vi "Engine-DI-Run.vi"(8 "Error In":errorcluster, 11 "DSI Reference":refnum<class "DCM-DSI.lvclass">) -> (0 "Error Out":errorcluster, 3 "DSI Reference":refnum<class "DCM-DSI.lvclass">)   [LabVIEW 2016, in "DSI-RT.lvlib"]
uses:
  DSI-RT.lvlib
  Classes/DCM-DSI/DCM-DSI.lvclass
  Classes/DCM-DSI/Read DI-A Command.vi
  Classes/DCM-DSI/Read DI-B Command.vi
  Classes/DCM-DSI/Read Channels.vi
  Classes/DCM-DSI/Write DI-A Command.vi
  Classes/DCM-DSI/Write DI-B Command.vi
  Classes/DCM-DSI/Write Channels.vi
  <vilib>/addons/Software Calibration Management/xSCM/CalPoint.xnode
  <vilib>/addons/Software Calibration Management/xSCM/FaultPoint.xnode
  <vilib>/addons/Software Calibration Management/xSCM/ni_scm.dll
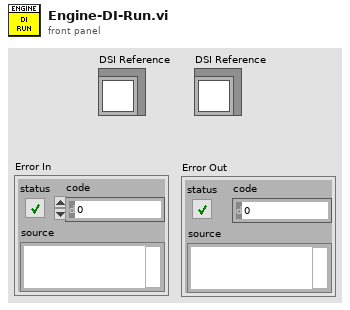
[diagram p1: front panel]
types:
  T1 = typedef "DCM - RT - DI.lvlib/Command.ctl" = cluster{"Mode":T2, "Digital Input":T3, "Default Profile Index":u8, "Cal Freq [Hz]":sgl, "Cal Duration [s]":sgl, "Cal Increment [s]":sgl, "Cal Pulses":u16, "TMP Command Sequence":T4[], "EPT TDC Offset [CAD]":sgl, "EPT Window Start [DBTDC]":sgl, "EPT Window End [DBTDC]":sgl, "EPT Angles":T5[], "EPT Skip Fire":bool, "EPT Skip Index":u8, "EPT Precharge Duration [s]":sgl, "EPT Precharge Profile Index":u8}
  T2 = typedef "DCM - FPGA - DI.lvlib/Mode.ctl" = enum8{"Off", "Direct", "Calibration", "Triggered Multi-Pulse", "Engine Position Tracking"}
  T3 = typedef "DCM - FPGA.lvlib/Digital Channel.ctl" = enum8{"Unused", "User OS", "Diff IO 1", "Diff IO 2", "Diff IO 3", "Diff IO 4", "Diff IO 5", "Diff IO 6", "Diff IO 7", "Diff IO 8", "Aux 1", "Aux 2", "Aux 3", "Aux 4", "Aux 5", "Aux 6", "Aux 7", "Aux 8", "Aux 9", "Aux 10", "Aux 11", "Aux 12", "Aux 13", "Aux 14", "Aux 15", "Aux 16"}
  T4 = typedef "DCM - RT - DI.lvlib/Command Sequence.ctl" = cluster{"Duration [s]":sgl, "Level":bool, "Run/Stop":bool, "Profile Index":u8}
  T5 = typedef "DCM - RT - DI.lvlib/Angle Control.ctl" = cluster{"Enable":bool, "Timing [DBTDC]":sgl, "Duration [s]":sgl, "Profile Index":u8}
  T6 = typedef "DCM-DSI.lvclass/Channel.ctl" = cluster{"Name":string, "Unit":string, "Value":sgl}
  T7 = typedef "DSI-Shared.lvlib/Engine-Channel.ctl" = cluster{"Name":string, "Unit":string, "Value":sgl}
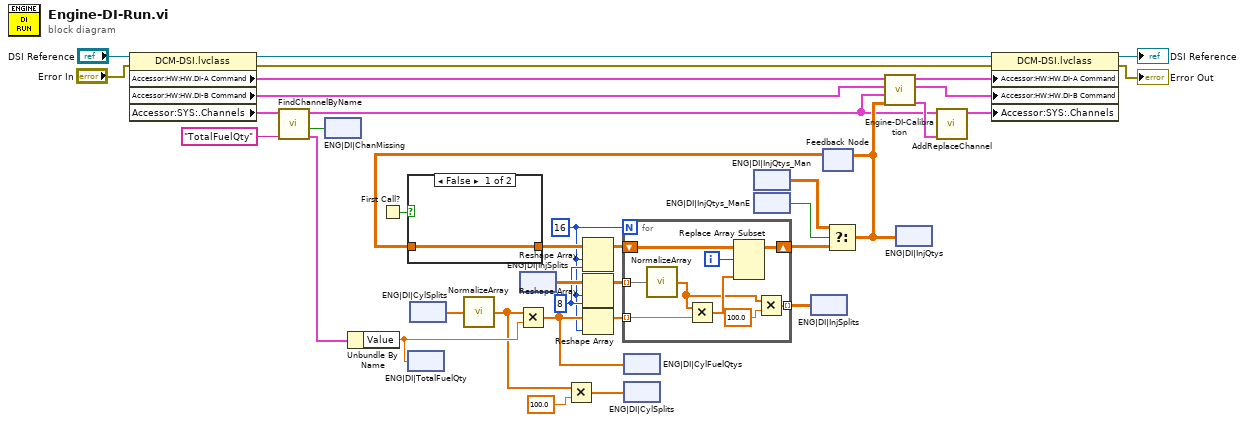
[diagram p0: block diagram]
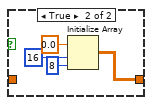
[diagram p2: hidden frame]
diagram:
  w13 = 8
  w12 = 16
  n1 = property class="DCM-DSI.lvclass"(reference="DSI Reference", error in="Error In") -> (reference out=w36:refnum<class "DCM-DSI.lvclass">, error out=w35:errorcluster, "Accessor:HW:HW.DI-A Command"=w30:T1[], "Accessor:HW:HW.DI-B Command"=w29:T1[], "Accessor:SYS:.Channels"=w10:T6[])
  n2 = call "FindChannelByName.vi"("Name"="TotalFuelQty", "CTRL.Channels in"=w10) -> ("Channel"=w9:T7, "Searching"=w1:bool, "CTRL.Channels out"=w6:T7[])  [unwired: 7 in]
  n3 = xnode "ENG|DI|ChanMissing"("Fault"=w1) -> ()
  n4 = Unbundle By Name(w9) -> ("Value"=w15:sgl)
  n5 = First Call?() -> (First Call?: T/F=w16:bool)
  n6 = xnode "ENG|DI|TotalFuelQty"("Value"=w15) -> ()
  n7 = xnode "ENG|DI|CylSplits"() -> ("Value"=w26:sgl[])
  n8 = call "NormalizeArray.vi"("Fuel Splits"=w26) -> ("Normalized Fuel Splits"=w5:sgl[])
  n9 = Multiply(x=w5, y=w15) -> (x*y=w22:sgl[])
  n10 = xnode "ENG|DI|InjSplits"() -> ("Value"=w27:sgl[][])
  n11 = Multiply(x=w5, y=sgl 100.0) -> (x*y=w4:sgl[])
  n12 = Reshape Array(w27, w12, w13) -> (w21:sgl[][])
  n13 = Reshape Array(w22, w12) -> (w20:sgl[])
  n14 = xnode "ENG|DI|CylFuelQtys"("Value"=w22) -> ()
  n15 = xnode "ENG|DI|CylSplits"("Value"=w4) -> ()
  n16 = xnode "ENG|DI|InjQtys_Man"() -> ("Value"=w23:sgl[][])
  n17 = xnode "ENG|DI|InjQtys_ManE"() -> ("Value"=w24:bool)
  n18 = feedback #1() -> (w18:sgl[][])  [unwired: 1 in]
  n19 = case shown="False" w16 {
    tunnel: [w38 w39] -> w17
    tunnel: w18 -> [w38 _]
    frame False {
    }
    frame True {
      n20 = Initialize Array(sgl 0.0 ("element"), 16 ("dimension size"), 8 ("dimension size")) -> (w39:sgl[][])
    }
  }
  n21 = Reshape Array(w17, w12, w13) -> (w14:sgl[][])
  n22 = for {
    N: w12 -> [_]
    tunnel: w21 -> [w48] mode=indexing
    shift-right: [w50] -> w25
    shift-left: w14 -> [w51]
    tunnel: w20 -> [w47] mode=indexing
    tunnel: [w43] -> w2 mode=indexing
    i -> [w46]
    n23 = call "NormalizeArray.vi"("Fuel Splits"=w48) -> ("Normalized Fuel Splits"=w44:sgl[])
    n24 = Multiply(x=w44, y=w47) -> (x*y=w49:sgl[])
    n25 = Replace Array Subset(array=w51, new element=w49, index (row)=w46) -> (w50:sgl[][])  [unwired: 1 in]
    n26 = Multiply(x=w44, y=sgl 100.0) -> (x*y=w43:sgl[])
  }
  n27 = xnode "ENG|DI|InjSplits"("Value"=w2) -> ()
  n28 = Select(t=w23, s=w24, f=w25) -> (s? t:f=w19:sgl[][])
  n29 = feedback-in #1(w19) -> ()
  n30 = call "Engine-DI-Calibration.vi"("Fueling"=w19, "Channels"=w6, "DI-B Command in"=w29, "DI-A Command in"=w30) -> ("DI.FuelQty"=w7:T7[], "DI-B Command out"=w31:T1[], "DI-A Command out"=w32:T1[])  [unwired: 5 in]
  n31 = xnode "ENG|DI|InjQtys"("Value"=w19) -> ()
  n32 = call "AddReplaceChannel.vi"("Channel In"=w7, "Channels in"=w6) -> ("Channels out"=w8:T7[])  [unwired: 9 in]
  n33 = property class="DCM-DSI.lvclass"(reference=w36, error in=w35, "Accessor:HW:HW.DI-A Command"=w32, "Accessor:HW:HW.DI-B Command"=w31, "Accessor:SYS:.Channels"=w8) -> (reference out=→"DSI Reference":refnum<class "DCM-DSI.lvclass">, error out=→"Error Out":errorcluster)
